vi "PPMS.MessageToProcess.vi"(6 "ID":string, 8 "error in (no error)":errorcluster, 9 "Data":variant, 10 "Command":string, 11 "instrument.PPMS in":refnum<class "instrument.PPMS.lvclass">) -> (0 "error out":errorcluster, 3 "instrument.PPMS out":refnum<class "instrument.PPMS.lvclass">)   [LabVIEW 2019, in "instrument.PPMS.lvclass"]
uses:
  instrument.PPMS.lvclass
  Typedefs/Private Events--MessageToProcess.ctl
  <userlib>/LevyLab/RemoteControl/Typedefs/Message--Cluster.ctl
  instrument.PPMS.lvclass/instrument.PPMS.ctl
  <userlib>/LevyLab/RemoteControl/RemoteControl.lvclass
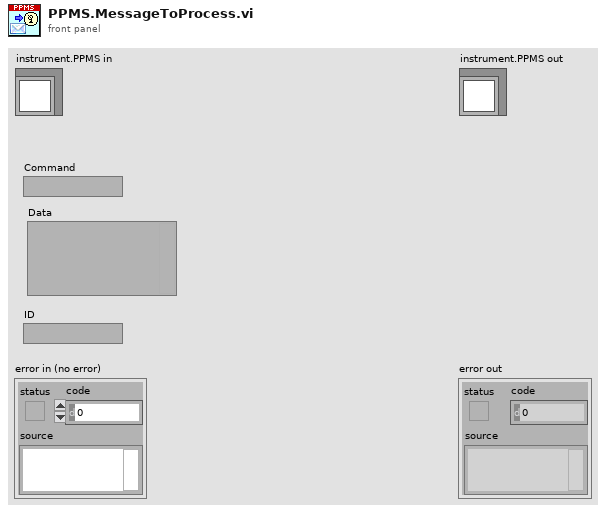
[diagram p1: front panel]
types:
  T1 = typedef "instrument.PPMS.lvclass/Private Events--MessageToProcess.ctl" = cluster{"Message":T2}
  T2 = typedef "RemoteControl.lvclass/Message--Cluster.ctl" = cluster{"Command":string, "Data":variant, "ID":string}
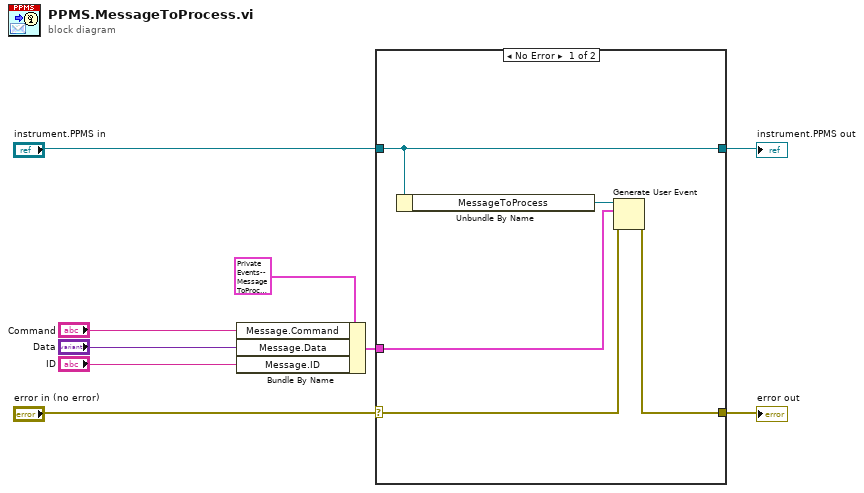
[diagram p0: block diagram]
diagram:
  n1 = Bundle By Name(cluster=T1 {"Message"={"Command"="", "Data"=variant(string ""), "ID"=""}} ("MessageToChildProcess"), "Message.Command"="Command", "Message.Data"="Data", "Message.ID"="ID") -> (w9:T1)
  n2 = case shown="No Error" "error in (no error)" {
    selector: "error in (no error)" -> [w14 w16]
    tunnel: [w12 w16] -> w1
    tunnel: [w11 w15] -> w3
    tunnel: "instrument.PPMS in" -> [w11 w15]
    tunnel: w9 -> [w10 _]
    frame No Error {
      n3 = Unbundle By Name(w11) -> ("MessageToProcess"=w13:refnum<user-event>)
      n4 = Generate User Event(user event=w13, event data cluster=w10, error in=w14) -> (error out=w12:errorcluster)  [unwired: 1 in, 1 out]
    }
    frame Error {
    }
  }
  "error out" <- w1
  "instrument.PPMS out" <- w3
